vi "Configure Single Pulse By Amplitude.vi"(0 "VISA resource name":refnum<visa-resource-name>="PG-AT", 5 "amplitude (0.01 V)":dbl=0.01 min=0.01 max=5.0, 7 "pulse width (s)":dbl=1e-09 min=0.005 max=5.0, 9 "offset (0V)":dbl min=0.005 max=5.0, 11 "error in (no error)":errorcluster, 12 "channel":i32=1 min=1 max=4) -> (4 "VISA resource name out":refnum<visa-resource-name>="PG-AT", 15 "error out":errorcluster)   [LabVIEW 2019, in "Pulse Rider PG-1000.lvlib"]
doc: "Configure the pulse generator to send a pulse with the characteristics given in parameters. The pulse will be between ``offset`` and ``amplitude``. The function will configure the right polarity \n\nThe pulse generator must be already configure in single mode and with the wanted delay and impedance.\n\namplitude: the pulse amplitude in V\nwidth: the pulse width in s\noffset: the amplitude offset in V\nchannel: the output channel int from 1 to 4"
uses:
  <instrlib>/LV_PulseRiderPG1000/Pulse Rider PG-1000.lvlib
  <instrlib>/LV_PulseRiderPG1000/Public/Configure/Pulse/Polarity.ctl
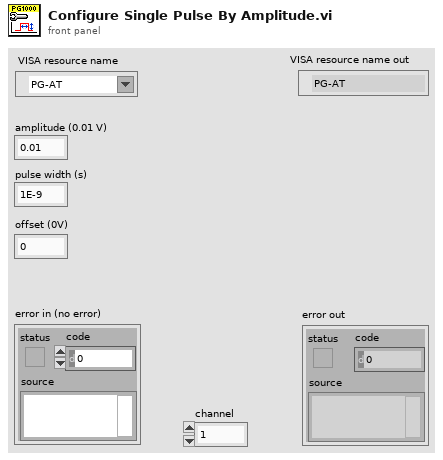
[diagram p1: front panel]
types:
  T1 = typedef "Pulse Rider PG-1000.lvlib/Polarity.ctl" = u16
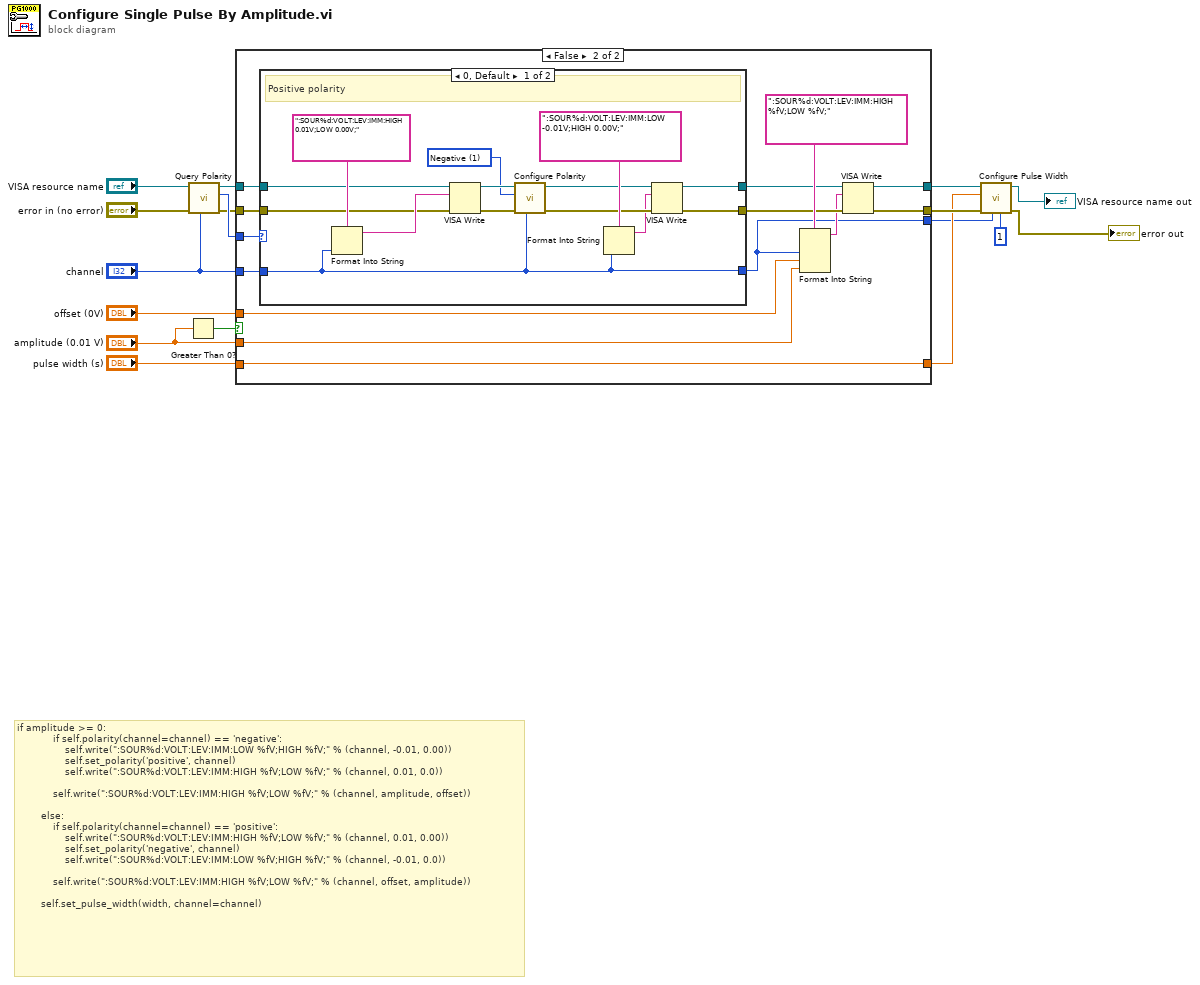
[diagram p0: block diagram]
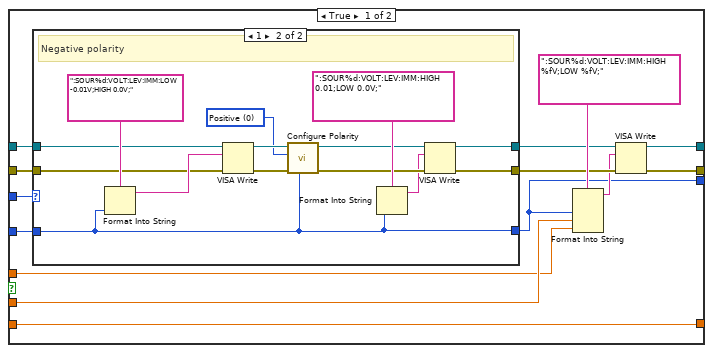
[diagram p2: hidden frame]
diagram:
  # "if amplitude >= 0:\n            if self.polarity(channel=channel) == 'negative':\n                self.write(\":SOUR%d:VOLT:LEV:IMM:LOW %fV;HIGH %fV;\" % (channel, -0.01, 0.00))\n                self.set_polarity('positive', channel)\n                self.write(\":SOUR%d:VOLT:LEV:IMM:HIGH %fV;LOW %fV;\" % (channel, 0.01, 0.0))\n\n            self.write(\":SOUR%d:VOLT:LEV:IMM:HIGH %fV;LOW %fV;\" % (channel, amplitude, offset))\n\n        else:\n            if self.polarity(channel=channel) == 'positive':\n                self.write(\":SOUR%d:VOLT:LEV:IMM:HIGH %fV;LOW %fV;\" % (channel, 0.01, 0.00))\n                self.set_polarity('negative', channel)\n                self.write(\":SOUR%d:VOLT:LEV:IMM:LOW %fV;HIGH %fV;\" % (channel, -0.01, 0.0))\n\n            self.write(\":SOUR%d:VOLT:LEV:IMM:HIGH %fV;LOW %fV;\" % (channel, offset, amplitude))\n\n        self.set_pulse_width(width, channel=channel)"
  n1 = Greater Than 0?(x="amplitude (0.01 V)") -> (x > 0?=w17:bool)
  n2 = call <instrlib>:"Query Polarity.vi"("channel"="channel", "error in (no error)"="error in (no error)", "VISA resource name"="VISA resource name") -> ("error out"=w12:errorcluster, "polarity"=w15:T1, "VISA resource name out"=w13:refnum<visa-resource-name>)  [unwired: 6 in]
  n3 = case shown="False" w17 {
    tunnel: w15 -> [w31 w62]
    tunnel: "channel" -> [w30 w61]
    tunnel: w13 -> [w29 w60]
    tunnel: w12 -> [w28 w59]
    tunnel: "amplitude (0.01 V)" -> [w23 w50]
    tunnel: "pulse width (s)" -> [w19 w52]
    tunnel: [w22 w54] -> w8
    tunnel: [w21 w53] -> w7
    tunnel: "offset (0V)" -> [w20 w51]
    tunnel: [w19 w52] -> w5
    tunnel: [w18 w49] -> w2
    frame True {
      n4 = case shown="1" w31 {
        tunnel: w30 -> [w32 w35]
        tunnel: w29 -> [w34 w46]
        tunnel: w28 -> [w33 w45]
        tunnel: [w34 w37] -> w26
        tunnel: [w33 w36] -> w25
        tunnel: [w32 w35] -> w18
        frame 0, Default {
          # "Positive polarity"
        }
        frame 1 {
          w42 = T1 0 items=["Positive", "Negative"] ("Polarity (0: Positive)")
          # "Negative polarity"
          n5 = Format Into String(format string=":SOUR%d:VOLT:LEV:IMM:LOW -0.01V;HIGH 0.0V;", w35) -> (resulting string=w47:string)  [unwired: 2 in, 1 out]
          n6 = VISA Write(VISA resource name=w46, write buffer=w47, error in (no error)=w45) -> (VISA resource name out=w44:refnum<visa-resource-name>, error out=w43:errorcluster)  [unwired: 1 out]
          n7 = call <instrlib>:"Configure Polarity.vi"("channel (1)"=w35, "error in (no error)"=w43, "Polarity (0: Positive)"=w42, "VISA resource name"=w44) -> ("error out"=w40:errorcluster, "VISA resource name out"=w39:refnum<visa-resource-name>)  [unwired: 6 in]
          n8 = Format Into String(format string=":SOUR%d:VOLT:LEV:IMM:HIGH 0.01;LOW 0.0V;", w35) -> (resulting string=w38:string)  [unwired: 2 in, 1 out]
          n9 = VISA Write(VISA resource name=w39, write buffer=w38, error in (no error)=w40) -> (VISA resource name out=w37:refnum<visa-resource-name>, error out=w36:errorcluster)  [unwired: 1 out]
        }
      }
      n10 = Format Into String(format string=":SOUR%d:VOLT:LEV:IMM:HIGH %fV;LOW %fV;", w18, w23, w20) -> (resulting string=w24:string)  [unwired: 2 in, 1 out]
      n11 = VISA Write(VISA resource name=w26, write buffer=w24, error in (no error)=w25) -> (VISA resource name out=w22:refnum<visa-resource-name>, error out=w21:errorcluster)  [unwired: 1 out]
    }
    frame False {
      n12 = case shown="0, Default" w62 {
        tunnel: w61 -> [w63 w77]
        tunnel: w60 -> [w74 w79]
        tunnel: w59 -> [w73 w78]
        tunnel: [w65 w79] -> w57
        tunnel: [w64 w78] -> w56
        tunnel: [w63 w77] -> w49
        frame 0, Default {
          w70 = T1 1 items=["Positive", "Negative"] ("Polarity (0: Positive)")
          # "Positive polarity"
          n13 = Format Into String(format string=":SOUR%d:VOLT:LEV:IMM:HIGH 0.01V;LOW 0.00V;", w63) -> (resulting string=w75:string)  [unwired: 2 in, 1 out]
          n14 = VISA Write(VISA resource name=w74, write buffer=w75, error in (no error)=w73) -> (VISA resource name out=w72:refnum<visa-resource-name>, error out=w71:errorcluster)  [unwired: 1 out]
          n15 = call <instrlib>:"Configure Polarity.vi"("channel (1)"=w63, "error in (no error)"=w71, "Polarity (0: Positive)"=w70, "VISA resource name"=w72) -> ("error out"=w68:errorcluster, "VISA resource name out"=w67:refnum<visa-resource-name>)  [unwired: 6 in]
          n16 = Format Into String(format string=":SOUR%d:VOLT:LEV:IMM:LOW -0.01V;HIGH 0.00V;", w63) -> (resulting string=w66:string)  [unwired: 2 in, 1 out]
          n17 = VISA Write(VISA resource name=w67, write buffer=w66, error in (no error)=w68) -> (VISA resource name out=w65:refnum<visa-resource-name>, error out=w64:errorcluster)  [unwired: 1 out]
        }
        frame 1 {
          # "Negative polarity"
        }
      }
      n18 = Format Into String(format string=":SOUR%d:VOLT:LEV:IMM:HIGH %fV;LOW %fV;", w49, w51, w50) -> (resulting string=w55:string)  [unwired: 2 in, 1 out]
      n19 = VISA Write(VISA resource name=w57, write buffer=w55, error in (no error)=w56) -> (VISA resource name out=w54:refnum<visa-resource-name>, error out=w53:errorcluster)  [unwired: 1 out]
    }
  }
  n20 = call <instrlib>:"Configure Pulse Width.vi"("pulse number"=1, "channel"=w2, "error in (no error)"=w7, "pulse width (s)"=w5, "VISA resource name"=w8) -> ("error out"=→"error out":errorcluster, "VISA resource name out"=→"VISA resource name out":refnum<visa-resource-name>)  [unwired: 5 in]
